vi "Dashboard Main.vi"() -> (0 "Camera Image":T3(plugin-control))   [LabVIEW 2011]
uses:
  <vilib>/Rock Robotics/WPI/Camera/WPI_CameraImageSize.ctl
  <vilib>/Rock Robotics/WPI/DriverStation/WPI_DriverStationDigitalData.ctl
panel:
  out "Target Info":T1(array[cluster])
  in  "Viewer":T2(tab)
  in  "Video Enable":bool=TRUE
  out "Processed Image":T3(plugin-control)
  in  "Range":cluster{"Lower value":sgl, "Upper value":sgl}={"Lower value"=234.67392, "Upper value"=255.0} {"Lower value" scale=0.0..255.0; "Upper value" scale=0.0..255.0}
  in  "Image Size":T4
  in  "1":bool
  in  "2":bool
  in  "3":bool
  in  "4":bool
  out "Position (From Selected)":cluster{"X":dbl, "Y":dbl}
  out "Buttons 1":cluster{"1":bool, "2":bool, "3":bool}
  out "Kinect 1":cluster{"X":dbl, "Y":dbl, "Z":dbl} {"X" scale=1.0..-1.0; "Y" scale=1.0..-1.0; "Z" scale=1.0..-1.0}
  out "Buttons 2":cluster{"1":bool, "2":bool, "3":bool}
  out "Kinect 2":cluster{"X":dbl, "Y":dbl, "Z":dbl} {"X" scale=1.0..-1.0; "Y" scale=1.0..-1.0; "Z" scale=1.0..-1.0}
  out "Version":string
  out "Skeleton Picture":picture
  out "Players":i8
  out "Dashboard Datatype Warning":string="Warning: The Dashboard Datatype used by the robot project and this dashboard do not match.\nSee diagram for more details."
  out "Image Error Message":string="Timeout in Camera Communications"
  # "1"
  # "2"
  # "3"
  # "4"
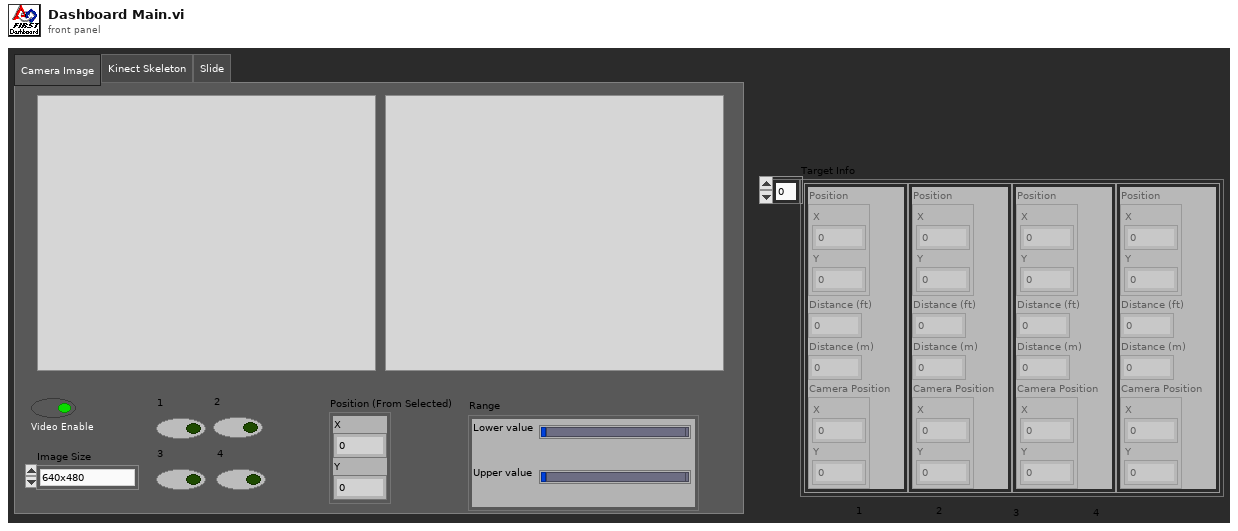
[diagram p1: front panel]
types:
  T1 = cluster{"Position":cluster{"X":dbl, "Y":dbl}, "Distance (ft)":dbl, "Distance (m)":dbl, "Camera Position":cluster{"X":dbl, "Y":dbl}}[]
  T2 = enum32{"Camera Image", "Kinect Skeleton", "Slide"}
  T3 = typedef "IMAQ Image.ctl" = refnum<image>
  T4 = typedef "WPI_CameraImageSize.ctl" = enum16{"640x480", "320x240", "160x120"}
  T5 = typedef "WPI_DriverStationDigitalData.ctl" = cluster{"Relay Fwd":u8, "Relay Rev":u8, "GPIO":u16, "GPIO_OE":u16, "PWM":cluster{"PWM[0]":u8, "PWM[1]":u8, "PWM[2]":u8, "PWM[3]":u8, "PWM[4]":u8, "PWM[5]":u8, "PWM[6]":u8, "PWM[7]":u8, "PWM[8]":u8, "PWM[9]":u8}}
  T6 = cluster{cluster{"AnalogModule[0]":cluster{"Channel[0]":sgl, "Channel[1]":sgl, "Channel[2]":sgl, "Channel[3]":sgl, "Channel[4]":sgl, "Channel[5]":sgl, "Channel[6]":sgl, "Channel[7]":sgl}, "AnalogModule[1]":cluster{"Channel[0]":sgl, "Channel[1]":sgl, "Channel[2]":sgl, "Channel[3]":sgl, "Channel[4]":sgl, "Channel[5]":sgl, "Channel[6]":sgl, "Channel[7]":sgl}}, cluster{"DigitalModule[0]":T5, "DigitalModule[1]":T5}, "Solenoid":u8}
  T7 = typedef "Image Type" = u32
  T8 = typedef "LVRectTypeDef.ctl" = cluster{"left":i16, "top":i16, "right":i16, "bottom":i16}
  T9 = typedef "SkeletonTrackState.ctl" = enum32{"NotTracked", "PositionOnly", "Tracked"}
  T10 = cluster{"TrackingState":u8[], "Position":cluster{"x":sgl, "y":sgl, "z":sgl}, cluster{"x":sgl, "y":sgl, "z":sgl, sgl}[], "TrackState":T9}
  T11 = cluster{cluster{"ScaledToPercentRange":dbl, "ScaledToPercentRange":dbl, "ScaledToPercentRange":dbl}, cluster{bool, bool, bool}}[]
  T12 = typedef "LVBoundsTypeDef.ctl" = cluster{"Width":u32, "Height":u32}
  T13 = cluster{cluster{"ScaledToPercentRange":dbl, "ScaledToPercentRange":dbl, "ScaledToPercentRange":dbl}, cluster{bool, bool, bool}}
  T14 = cluster{"ScaledToPercentRange":dbl, "ScaledToPercentRange":dbl, "ScaledToPercentRange":dbl}
  T15 = cluster{"Competition mode":bool, "Robot Link":bool, "Autonomous":bool, "Enabled":bool, "E-Stop":bool}
  T16 = cluster{"AnalogModule[0]":cluster{"Channel[0]":sgl, "Channel[1]":sgl, "Channel[2]":sgl, "Channel[3]":sgl, "Channel[4]":sgl, "Channel[5]":sgl, "Channel[6]":sgl, "Channel[7]":sgl}, "AnalogModule[1]":cluster{"Channel[0]":sgl, "Channel[1]":sgl, "Channel[2]":sgl, "Channel[3]":sgl, "Channel[4]":sgl, "Channel[5]":sgl, "Channel[6]":sgl, "Channel[7]":sgl}}
  T17 = cluster{"DigitalModule[0]":T5, "DigitalModule[1]":T5}
  T18 = cluster{"Channel[0]":sgl, "Channel[1]":sgl, "Channel[2]":sgl, "Channel[3]":sgl, "Channel[4]":sgl, "Channel[5]":sgl, "Channel[6]":sgl, "Channel[7]":sgl}[]
  T19 = cluster{"Channel[0]":sgl, "Channel[1]":sgl, "Channel[2]":sgl, "Channel[3]":sgl, "Channel[4]":sgl, "Channel[5]":sgl, "Channel[6]":sgl, "Channel[7]":sgl}
  T20 = cluster{"fps":i32, "compression":i32, "Image Size":T4}
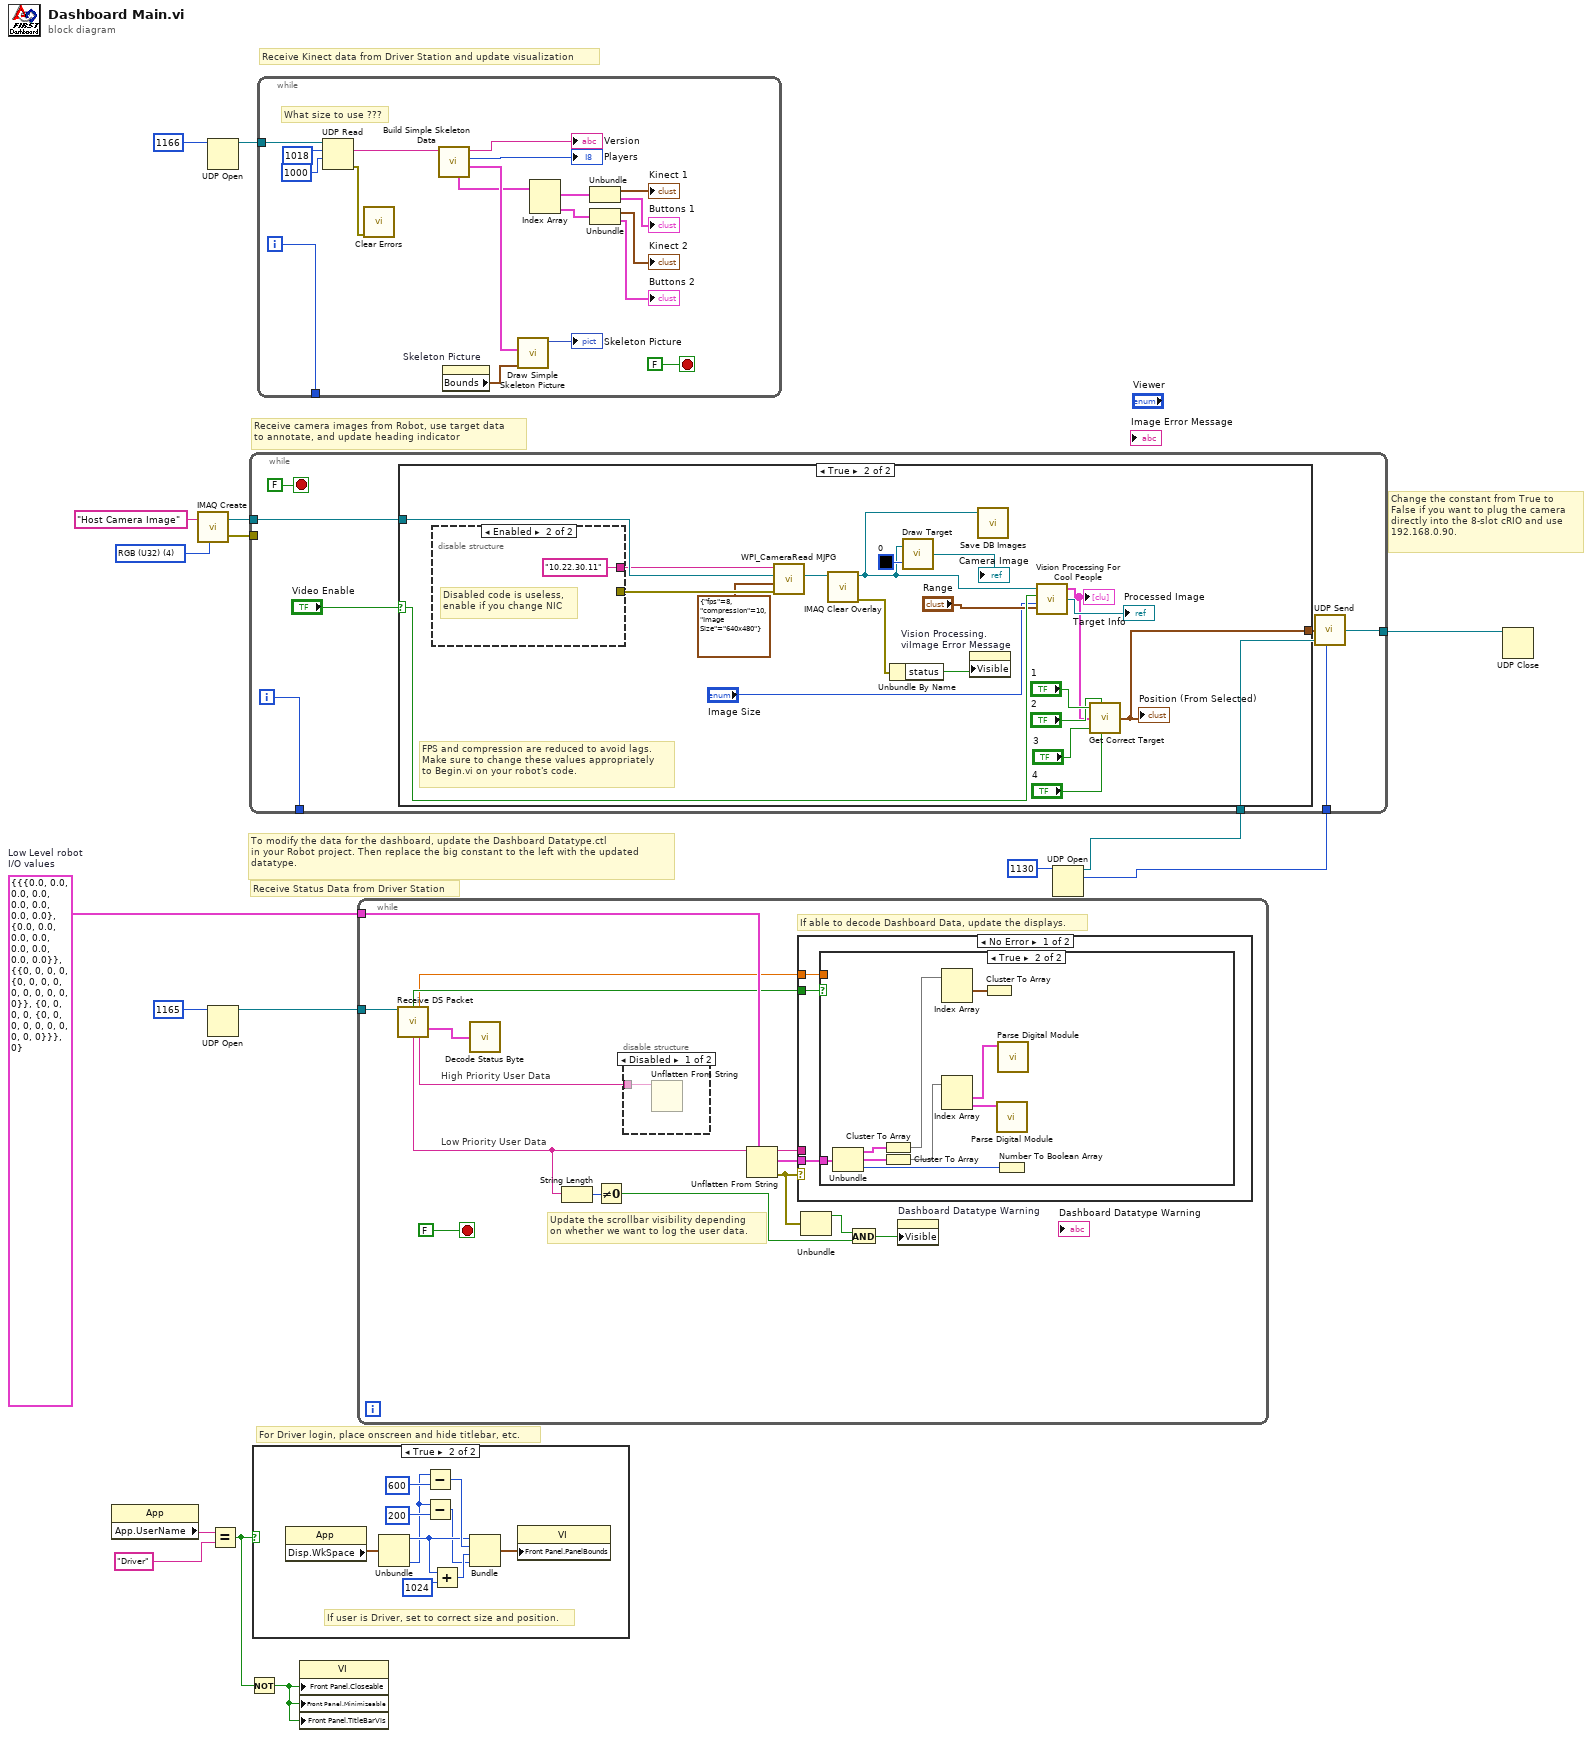
[diagram p0: block diagram]
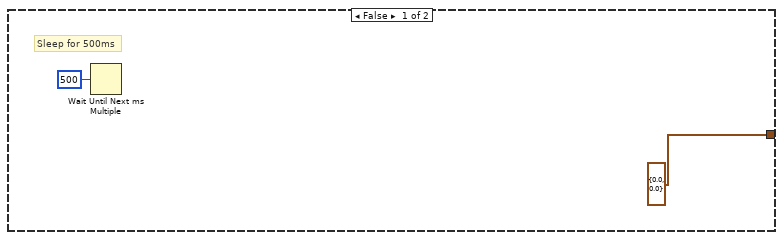
[diagram p6: hidden frame]
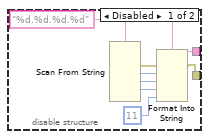
[diagram p7: hidden frame]
diagram:
  w7 = T6 {{"AnalogModule[0]"={"Channel[0]"=0.0, "Channel[1]"=0.0, "Channel[2]"=0.0, "Channel[3]"=0.0, "Channel[4]"=0.0, "Channel[5]"=0.0, "Channel[6]"=0.0, "Channel[7]"=0.0}, "AnalogModule[1]"={"Channel[0]"=0.0, "Channel[1]"=0.0, "Channel[2]"=0.0, "Channel[3]"=0.0, "Channel[4]"=0.0, "Channel[5]"=0.0, "Channel[6]"=0.0, "Channel[7]"=0.0}}, {"DigitalModule[0]"={"Relay Fwd"=0, "Relay Rev"=0, "GPIO"=0, "GPIO_OE"=0, "PWM"={"PWM[0]"=0, "PWM[1]"=0, "PWM[2]"=0, "PWM[3]"=0, "PWM[4]"=0, "PWM[5]"=0, "PWM[6]"=0, "PWM[7]"=0, "PWM[8]"=0, "PWM[9]"=0}}, "DigitalModule[1]"={"Relay Fwd"=0, "Relay Rev"=0, "GPIO"=0, "GPIO_OE"=0, "PWM"={"PWM[0]"=0, "PWM[1]"=0, "PWM[2]"=0, "PWM[3]"=0, "PWM[4]"=0, "PWM[5]"=0, "PWM[6]"=0, "PWM[7]"=0, "PWM[8]"=0, "PWM[9]"=0}}}, "Solenoid"=0}  # Low Level robot I/O values
  w15 = T7 4 items=["Grayscale (U8)", "Grayscale (I16)", "Grayscale (SGL)", "Complex (CSG)", "RGB (U32)", "HSL (U32)", "RGB (U64)"] ("Image Type")
  # "Change the constant from True to\nFalse if you want to plug the camera\ndirectly into the 8-slot cRIO and use\n192.168.0.90."
  # "Receive Kinect data from Driver Station and update visualization"
  # "For Driver login, place onscreen and hide titlebar, etc."
  # "To modify the data for the dashboard, update the Dashboard Datatype.ctl\nin your Robot project. Then replace the big constant to the left with the updated\ndatatype."
  # "Receive Status Data from Driver Station"
  # "Receive camera images from Robot, use target data\nto annotate, and update heading indicator"
  n1 = property class="App"() -> ("App.UserName"=w10:string)  [unwired: 2 in, 2 out]
  n2 = call "IMAQ Create"("Image Name"="Host Camera Image", "Image Type"=w15) -> ("New Image"=w13:T3, "error out"=w12:errorcluster)  [unwired: 2 in, 1 out]
  n3 = UDP Open(11:u16 1166 ("port")) -> (port=w5:refnum<k16>)  [unwired: 2 in, 4 out]
  n4 = UDP Open(11:u16 1165 ("port")) -> (port=w16:refnum<k16>)  [unwired: 2 in, 4 out]
  n5 = Equal?(x=w10, y="Driver") -> (x = y?=w9:bool)
  n6 = Not(x=w9) -> (.not. x?=w8:bool)
  n7 = case shown="True" w9 {
    frame False {
    }
    frame True {
      # "If user is Driver, set to correct size and position."
      n8 = property class="App"() -> ("Disp.WkSpace"=w27:T8)  [unwired: 2 in, 2 out]
      n9 = Unbundle(w27) -> ("left"=w22:i16, "bottom"=w18:i16)  [unwired: 2 out]
      n10 = Subtract(x=w18, y=600) -> (x-y=w24:i32)
      n11 = Subtract(x=w18, y=200) -> (x-y=w19:i32)
      n12 = Add(x=w22, y=1024) -> (x+y=w23:i32)
      n13 = Bundle("left"=w22, w24, w23, w19) -> (w26:cluster{"left":i16, i32, i32, i32})  [unwired: 1 out]
      n14 = property class="VI"("Front Panel.PanelBounds"=w26) -> ()  [unwired: 2 in, 2 out]
    }
  }
  n15 = while {
    tunnel: w5 -> [w44]
    tunnel: [w28] -> _
    i -> [w28]
    stop <- FALSE stop-if-true
    # "What size to use ???"
    n16 = UDP Read(connection ID=w44, max size (548)=1018 ("bytes to read"), timeout ms (25000)=1000) -> (data out=w38:string, error out=w36:errorcluster)  [unwired: 1 in, 3 out]
    n17 = call <vilib>:"Clear Errors.vi"("error in (no error)"=w36) -> ()  [unwired: 6 in, 1 out]
    n18 = call "Build Simple Skeleton Data.vi"("data out"=w38) -> ("Skeleton Data"=w39:T10, "NumPlayers"=→"Players":i8, "Version String"=→"Version":string, "Simple Joystick Info"=w35:T11)  [unwired: 6 in, 1 out]
    n19 = property on="Skeleton Picture" class="Pict"() -> ("Bounds"=w40:T12)  [unwired: 2 in, 2 out]
    n20 = call "Draw Simple Skeleton Picture.vi"("Bounds"=w40, "Simple Skeleton"=w39) -> ("new picture out"=→"Skeleton Picture":picture)  [unwired: 9 in]
    n21 = Index Array(array=w35) -> (element #1=w34:T13, element #2=w33:T13)  [unwired: 2 in]
    n22 = Unbundle(w34) -> (→"Kinect 1":T14, →"Buttons 1":cluster{bool, bool, bool})
    n23 = Unbundle(w33) -> (→"Kinect 2":T14, →"Buttons 2":cluster{bool, bool, bool})
  }
  n24 = property class="VI"("Front Panel.Closeable"=w8, "Front Panel.Minimizeable"=w8, "Front Panel.TitleBarVis"=w8) -> ()  [unwired: 2 in, 2 out]
  n25 = while {
    tunnel: w16 -> [w59]
    tunnel: w7 -> [w58]
    stop <- FALSE stop-if-true
    # "High Priority User Data"
    # "Low Priority User Data"
    # "Update the scrollbar visibility depending\non whether we want to log the user data."
    # "If able to decode Dashboard Data, update the displays."
    n26 = call "Receive DS Packet.vi"("Recv Socket"=w59) -> ("New Dashboard Data"=w55:bool, "Battery"=w47:sgl, "Status"=w60:T15, "Low Priority User Data"=w49:string, "High Priority User Data"=w48:string)  [unwired: 1 in, 9 out]
    n27 = call "Decode Status Byte.vi"("Status Byte"=w60) -> ()  [unwired: 2 out]
    n28 = String Length(string=w49) -> (length=w50:i32)
    n29 = Not Equal To 0?(x=w50) -> (x != 0?=w53:bool)
    n30 = disable-structure shown="Disabled" {
      disable-tunnel: w48 -> [w62 _]
      frame Disabled {
        n31 = Unflatten From String(binary string=w62) -> ()  [unwired: 2 in, 5 out]
      }
      frame Enabled {
      }
    }
    n32 = Unflatten From String(type=w58, binary string=w49) -> (rest of the binary string=w51:string, value=w57:T6, error out=w56:errorcluster)  [unwired: 1 in, 2 out]
    n33 = case shown="No Error" w56 {
      tunnel: w57 -> [w65 _]
      tunnel: w55 -> [w64 _]
      tunnel: w51 -> [_ _]
      tunnel: w47 -> [w63 _]
      frame No Error {
        n34 = case shown="True" w64 {
          tunnel: w65 -> [_ w70]
          tunnel: w63 -> [_ _]
          frame False {
            # "Don't update if the robot hasn't sent new data"
          }
          frame True {
            n35 = Unbundle(w70) -> (w67:T16, w68:T17, "Solenoid"=w69:u8)
            n36 = Cluster To Array(cluster=w67) -> (array=w74:T18)
            n37 = Cluster To Array(cluster=w68) -> (array=w73:T5[])
            n38 = Index Array(array=w74) -> (element #1=w66:T19)  [unwired: 2 in, 1 out]
            n39 = Index Array(array=w73) -> (element #1=w72:T5, element #2=w71:T5)  [unwired: 2 in]
            n40 = Cluster To Array(cluster=w66) -> ()  [unwired: 1 out]
            n41 = call "Parse Digital Module.vi"("DigitalModule"=w71) -> ()  [unwired: 11 out]
            n42 = Number To Boolean Array(number=w69) -> ()  [unwired: 1 out]
            n43 = call "Parse Digital Module.vi"("DigitalModule"=w72) -> ()  [unwired: 11 out]
          }
        }
      }
      frame Error {
        # "Your datatypes don't match. The Dashboard Datatype.ctl in your Robot project\nand the big constant to the left of the loop need to match."
      }
    }
    n44 = Unbundle(w56) -> ("status"=w52:bool)  [unwired: 2 out]
    n45 = And(x=w52, y=w53) -> (x .and. y?=w54:bool)
    n46 = property on="Dashboard Datatype Warning" class="Str"("Visible"=w54) -> ()  [unwired: 2 in, 2 out]
  }
  n47 = UDP Open(11:u16 1130 ("port")) -> (port=w3:refnum<k16>, 2:w2:u16)  [unwired: 1 in, 4 out]
  n48 = while {
    tunnel: w13 -> [w81]
    tunnel: w12 -> [_]
    tunnel: [w79] -> _
    tunnel: w3 -> [w78]
    tunnel: w2 -> [w77]
    tunnel: [w76] -> w1
    i -> [w79]
    stop <- FALSE stop-if-true
    n49 = case shown="True" "Video Enable" {
      selector: "Video Enable" -> [_ w98]
      tunnel: w81 -> [_ w104]
      tunnel: [cluster{"X":dbl, "Y":dbl} {"X"=0.0, "Y"=0.0} ("Position") w85] -> w75
      frame False {
        # "Sleep for 500ms"
        n50 = Wait Until Next ms Multiple(millisecond multiple=u32 500) -> ()  [unwired: 1 out]
      }
      frame True {
        # "FPS and compression are reduced to avoid lags.\nMake sure to change these values appropriately\nto Begin.vi on your robot's code."
        n51 = disable-structure shown="Enabled" {
          disable-tunnel: [w108 "10.22.30.11" ("address")] -> w100
          disable-tunnel: [w107 _] -> w99
          frame Disabled {
            w105 = "%d.%d.%d.%d" ("format string")
            n52 = Scan From String(format string=w105) -> (error out=w109:errorcluster, output 1=w110:i32, output 2=w111:i32, output 3=w112:i32)  [unwired: 3 in, 7 out]
            n53 = Format Into String(format string=w105, error in=w109, w110, w111, w112, 11 ("IP Suffix:")) -> (resulting string=w108:string, error out=w107:errorcluster)  [unwired: 1 in]
          }
          frame Enabled {
            # "Disabled code is useless,\nenable if you change NIC"
          }
        }
        n54 = call <vilib>:"WPI_CameraRead MJPG.vi"("error in"=w99, "Camera Settings"=T20 {"fps"=8, "compression"=10, "Image Size"=enum."640x480"}, "Image"=w104, "address"=w100) -> ("Image Out"=w101:T3)  [unwired: 6 in, 1 out]
        n55 = call "IMAQ Clear Overlay"("Image"=w101) -> ("error out"=w102:errorcluster, "Image Out"=w86:T3)  [unwired: 2 in, 7 out]
        n56 = Unbundle By Name(w102) -> ("status"=w103:bool)
        n57 = call "Draw Target.vi"("Color"=u32 0, "Original Image"=w86) -> ("Image Out"=→"Camera Image":T3)
        n58 = property on="Vision Processing.viImage Error Message" class="Str"("Visible"=w103) -> ()  [unwired: 2 in, 2 out]
        n59 = call "Save DB Images.vi"("Image"=w86) -> ()  [unwired: 2 in, 1 out]
        n60 = call "Vision Processing For Cool People.vi"("Range"="Range", "Image Size"="Image Size", "View 2"=w98, "Original Image"=w86) -> ("Processed Image"=→"Processed Image":T3, "Target Info"=w89:T1)  [unwired: 1 out]
        "Target Info" <- w89
        n61 = call "Get Correct Target.vi"("1"="1", "2"="2", "Target Info"=w89, "3"="3", "4"="4") -> ("Position"=w85:cluster{"X":dbl, "Y":dbl})
        "Position (From Selected)" <- w85
      }
    }
    n62 = call "UDP Send.vi"("Cluster"=w75, "connection ID"=w78, "port"=w77) -> ("connection ID out"=w76:refnum<k16>)  [unwired: 2 in]
  }
  n63 = UDP Close(connection ID=w1) -> ()  [unwired: 1 in, 2 out]
